vi "array -- poor man hash table -- cluster keyed .vi"(0 "key table":T2[](array[typedef]), 1 "hash key":T2, 2 "value table":T1[](array[typedef]), 3 "torque -- hash value":T1={"time (sec) array"=[], "temperature (K) array"=[], "SRS Vx (V) array"=[], "field (T) array"=[], "filename"="name", "time OK?"=FALSE, "temperature OK?"=FALSE, "SRS OK?"=FALSE, "FIELD OK?"=FALSE}, 6 "hash action":T3) -> (14 "Key table OUT":T2[](array[typedef]), 15 "hash key OUT":T2, 16 "value table OUT":T1[](array[typedef]), 17 "torque -- hash value OUT":T1={"time (sec) array"=[], "temperature (K) array"=[], "SRS Vx (V) array"=[], "field (T) array"=[], "filename"="name", "time OK?"=FALSE, "temperature OK?"=FALSE, "SRS OK?"=FALSE, "FIELD OK?"=FALSE}, 18 "index":i32, 19 "found?":bool)   [LabVIEW 2012]
uses:
  hash action control.ctl
  torque -- hash key.ctl
  torque -- hash value.ctl
  stack action -- control.ctl
  hash status control.ctl
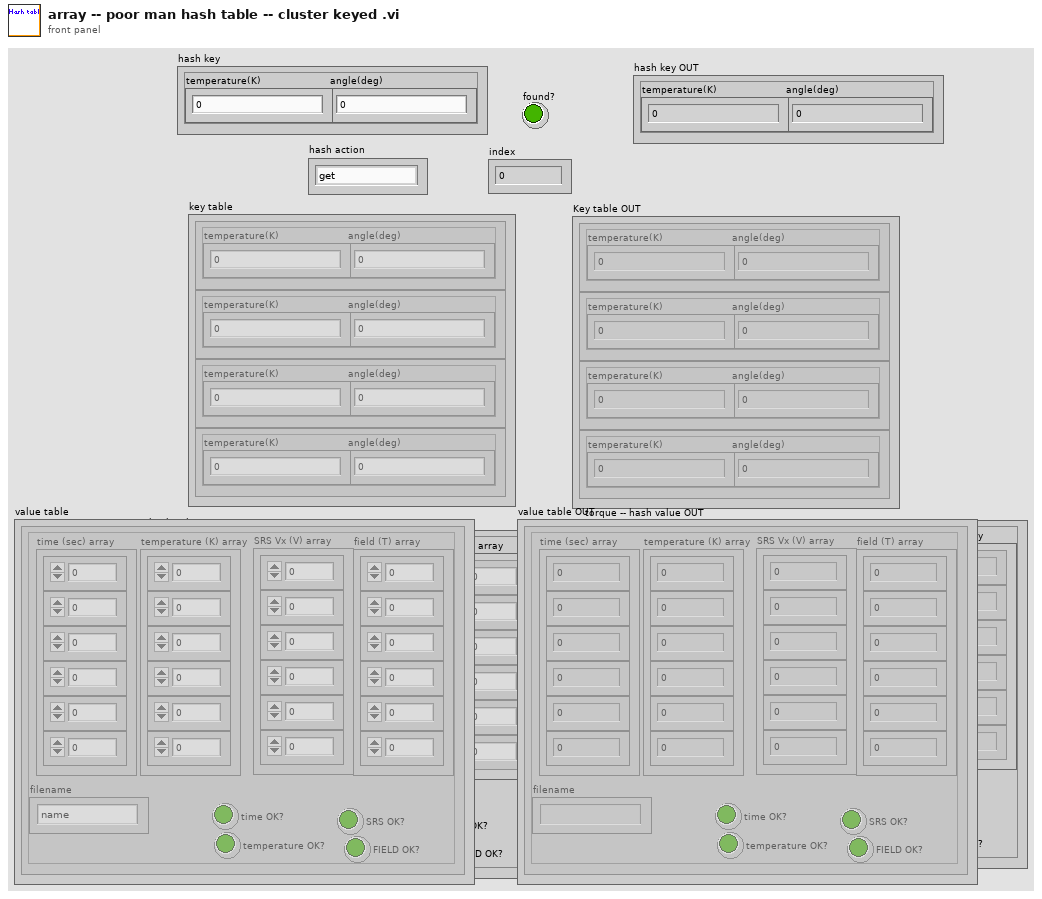
[diagram p1: front panel]
types:
  T1 = typedef "torque -- hash value.ctl" = cluster{"time (sec) array":dbl[], "temperature (K) array":dbl[], "SRS Vx (V) array":dbl[], "field (T) array":dbl[], "filename":string, "time OK?":bool, "temperature OK?":bool, "SRS OK?":bool, "FIELD OK?":bool}
  T2 = typedef "torque -- hash key.ctl" = cluster{"temperature(K)":dbl, "angle(deg)":dbl}
  T3 = typedef "hash action control.ctl" = enum16{"get", "new", "--void", "delete", "delete all", "set", "--delete if exists", "--create if not there", "list keys", "index forw", "index back", "check", "index set", "find key"}
  T4 = typedef "stack action -- control.ctl" = enum16{"push", "pop", "check", "init"}
  T5 = typedef "hash status control.ctl" = enum16{"exists", "does not exists"}
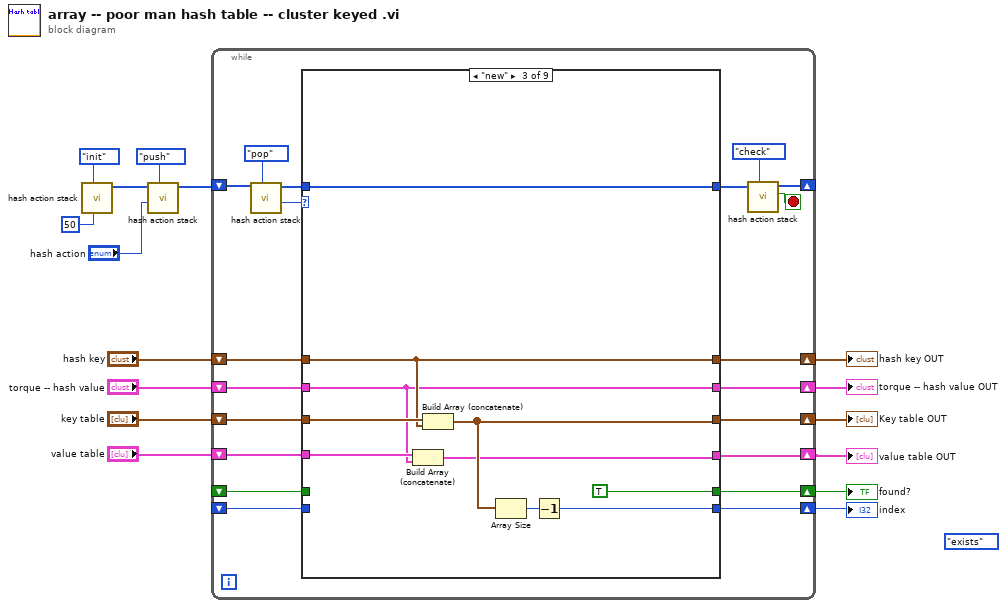
[diagram p0: block diagram]
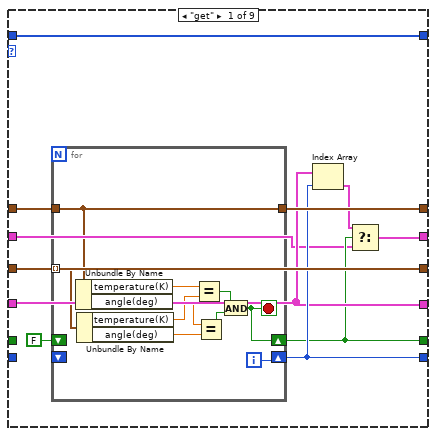
[diagram p2: hidden frame]
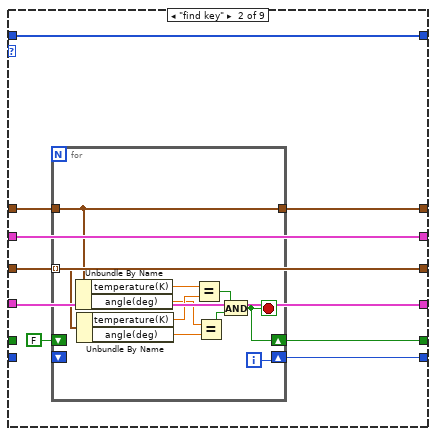
[diagram p3: hidden frame]
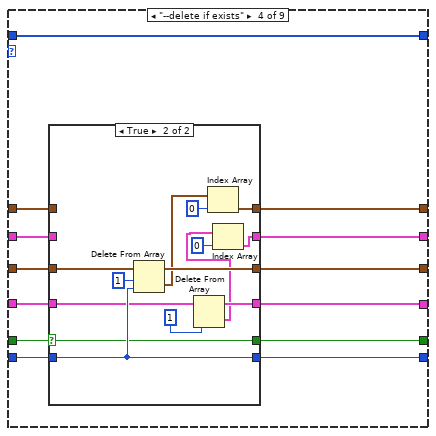
[diagram p4: hidden frame]
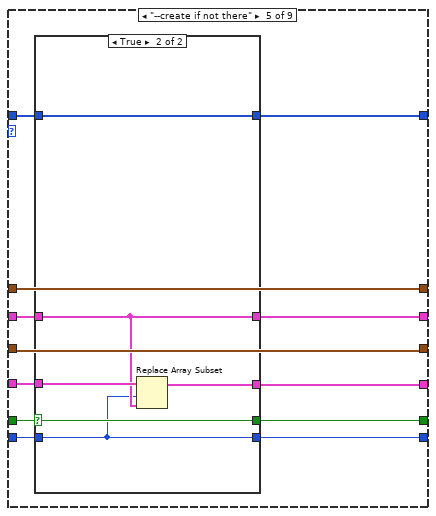
[diagram p6: hidden frame]
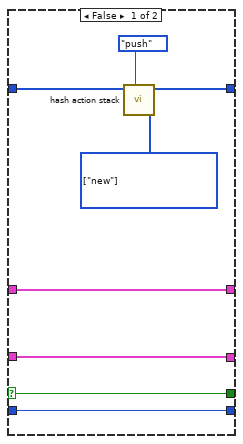
[diagram p7: hidden frame]
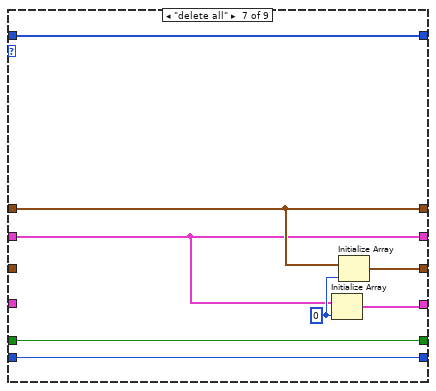
[diagram p9: hidden frame]
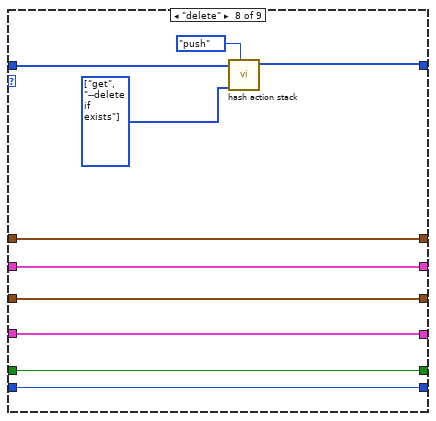
[diagram p10: hidden frame]
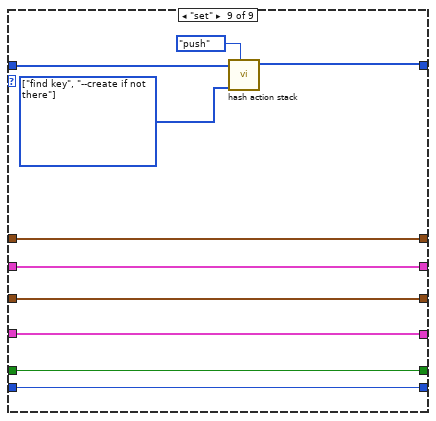
[diagram p11: hidden frame]
diagram:
  (unwired) hash_status_control."exists" ("hash status")
  n1 = call "hash action stack.vi"("init size"=50 ("dimension size"), "stack action"=stack_action_--_control."init") -> ("command stack out"=w12:T3[])  [unwired: 7 in, 2 out]
  n2 = call "hash action stack.vi"("stack action"=stack_action_--_control."push", "hash action"="hash action", "command stack"=w12) -> ("command stack out"=w14:T3[])  [unwired: 6 in, 2 out]
  n3 = while {
    shift-right: [w30] -> _
    shift-left: w14 -> [w29]
    shift-right: [w27] -> w9
    shift-left: _ -> [w21]
    shift-right: [w28] -> w10
    shift-left: _ -> [w22]
    shift-right: [w26] -> w8
    shift-left: "key table" -> [w23]
    shift-right: [w25] -> w7
    shift-left: "hash key" -> [w24]
    shift-right: [w20] -> w4
    shift-left: "torque -- hash value" -> [w18]
    shift-right: [w17] -> w3
    shift-left: "value table" -> [w19]
    stop <- w31 stop-if-true
    n4 = call "hash action stack.vi"("stack action"=stack_action_--_control."pop", "command stack"=w29) -> ("cursor window action out"=w32:T3, "command stack out"=w35:T3[])  [unwired: 7 in, 1 out]
    n5 = case shown="\"new\"" w32 {
      tunnel: w35 -> [w47 w66 w86 w99 w125 w152 w160 w164 w172]
      tunnel: [w47 w66 w86 w99 w124 w152 w160 w163 w171] -> w33
      tunnel: w23 -> [w43 w62 w85 w98 w126 w150 _ w169 w179]
      tunnel: w24 -> [w46 w65 w84 w91 w131 w151 w156 w170 w180]
      tunnel: [w40 w59 TRUE w93 w127 w149 w159 w168 w178] -> w28
      tunnel: [w42 w61 w81 w94 w128 w148 w158 w167 w177] -> w27
      tunnel: [w43 w62 w83 w97 w126 w150 w155 w169 w179] -> w26
      tunnel: [w44 w63 w84 w92 w131 w151 w156 w170 w180] -> w25
      tunnel: w22 -> [_ _ _ w95 w129 w149 w159 w168 w178]
      tunnel: w21 -> [_ _ _ w96 w130 w148 w158 w167 w177]
      tunnel: [w38 w58 w78 w90 w120 w147 w154 w162 w174] -> w20
      tunnel: w18 -> [w37 w58 w78 w89 w121 w147 w154 w162 w174]
      tunnel: w19 -> [w41 w60 w79 w87 w123 w146 _ w161 w173]
      tunnel: [w41 w60 w77 w88 w122 w146 w153 w161 w173] -> w17
      frame "get" {
        n6 = for {
          tunnel: w43 -> [w49] mode=indexing
          tunnel: w46 -> [w48]
          shift-right: [w51] -> w40
          shift-left: FALSE -> [_]
          shift-right: [w50] -> w42
          shift-left: _ -> [_]
          tunnel: [w48] -> w44
          i -> [w50]
          stop <- w51 stop-if-true
          n7 = Unbundle By Name(w48) -> ("temperature(K)"=w56:dbl, "angle(deg)"=w55:dbl)
          n8 = Unbundle By Name(w49) -> ("temperature(K)"=w57:dbl, "angle(deg)"=w54:dbl)
          n9 = Equal?(x=w56, y=w57) -> (x = y?=w53:bool)
          n10 = Equal?(x=w55, y=w54) -> (x = y?=w52:bool)
          n11 = And(x=w53, y=w52) -> (x .and. y?=w51:bool)
        }
        n12 = Index Array(array=w41, index=w42) -> (element=w39:T1)
        n13 = Select(t=w39, s=w40, f=w37) -> (s? t:f=w38:T1)
      }
      frame "find key" {
        n14 = for {
          tunnel: w62 -> [w68] mode=indexing
          tunnel: w65 -> [w67]
          shift-right: [w70] -> w59
          shift-left: FALSE -> [_]
          shift-right: [w69] -> w61
          shift-left: _ -> [_]
          tunnel: [w67] -> w63
          i -> [w69]
          stop <- w70 stop-if-true
          n15 = Unbundle By Name(w67) -> ("temperature(K)"=w75:dbl, "angle(deg)"=w74:dbl)
          n16 = Unbundle By Name(w68) -> ("temperature(K)"=w76:dbl, "angle(deg)"=w73:dbl)
          n17 = Equal?(x=w75, y=w76) -> (x = y?=w72:bool)
          n18 = Equal?(x=w74, y=w73) -> (x = y?=w71:bool)
          n19 = And(x=w72, y=w71) -> (x .and. y?=w70:bool)
        }
      }
      frame "new" {
        n20 = Build Array (concatenate)(w79, w78) -> (w77:T1[])
        n21 = Build Array (concatenate)(w85, w84) -> (w83:T2[])
        n22 = Array Size(array=w83) -> (size(s)=w82:i32)
        n23 = Decrement(x=w82) -> (x-1=w81:i32)
      }
      frame "--delete if exists" {
        n24 = case shown="True" w95 {
          selector: w95 -> [w104 w115]
          tunnel: w98 -> [w105 w119]
          tunnel: [w105 w118] -> w97
          tunnel: w96 -> [w103 w116]
          tunnel: [w103 w116] -> w94
          tunnel: [w104 w115] -> w93
          tunnel: [w102 w112] -> w92
          tunnel: w91 -> [w102 _]
          tunnel: [w101 w107] -> w90
          tunnel: w89 -> [w101 _]
          tunnel: [w100 w110] -> w88
          tunnel: w87 -> [w100 w109]
          frame False {
          }
          frame True {
            n25 = Delete From Array(array=w119, length=1, index=w116) -> (deleted portion=w114:T2[], array with subset deleted=w118:T2[])
            n26 = Delete From Array(array=w109, length=1) -> (deleted portion=w106:T1[], array with subset deleted=w110:T1[])  [unwired: 1 in]
            n27 = Index Array(array=w114, index=0) -> (element=w112:T2)
            n28 = Index Array(array=w106, index=0) -> (element=w107:T1)
          }
        }
      }
      frame "--create if not there" {
        n29 = case shown="True" w129 {
          selector: w129 -> [w138 w145]
          tunnel: w130 -> [w139 w140]
          tunnel: [w139 w140] -> w128
          tunnel: [w138 w145] -> w127
          tunnel: w125 -> [w136 w144]
          tunnel: [w135 w144] -> w124
          tunnel: w123 -> [w133 w143]
          tunnel: [w133 w142] -> w122
          tunnel: w121 -> [w134 w141]
          tunnel: [w134 w141] -> w120
          frame False {
            w132 = T3[] [enum."new"] items=["get", "new", "--void", "delete", "delete all", "set", "--delete if exists", "--create if not there", "list keys", "index forw", "index back", "check", "index set", "find key"] ("hash action list")
            n30 = call "hash action stack.vi"("stack action"=stack_action_--_control."push", "hash action list"=w132, "command stack"=w136) -> ("command stack out"=w135:T3[])  [unwired: 6 in, 2 out]
          }
          frame True {
            n31 = Replace Array Subset(array=w143, new element=w141, index=w140) -> (w142:T1[])
          }
        }
      }
      frame "--void", Default {
      }
      frame "delete all" {
        w157 = 0 ("dimension size")
        n32 = Initialize Array(w154, w157) -> (w153:T1[])
        n33 = Initialize Array(w156, w157) -> (w155:T2[])
      }
      frame "delete" {
        w165 = T3[] [enum."get", enum."--delete if exists"] items=["get", "new", "--void", "delete", "delete all", "set", "--delete if exists", "--create if not there", "list keys", "index forw", "index back", "check", "index set", "find key"] ("hash action list")
        n34 = call "hash action stack.vi"("stack action"=stack_action_--_control."push", "hash action list"=w165, "command stack"=w164) -> ("command stack out"=w163:T3[])  [unwired: 6 in, 2 out]
      }
      frame "set" {
        w175 = T3[] [enum."find key", enum."--create if not there"] items=["get", "new", "--void", "delete", "delete all", "set", "--delete if exists", "--create if not there", "list keys", "index forw", "index back", "check", "index set", "find key"] ("hash action list")
        n35 = call "hash action stack.vi"("stack action"=stack_action_--_control."push", "hash action list"=w175, "command stack"=w172) -> ("command stack out"=w171:T3[])  [unwired: 6 in, 2 out]
      }
    }
    n36 = call "hash action stack.vi"("stack action"=stack_action_--_control."check", "command stack"=w33) -> ("stack is empty ?"=w31:bool, "command stack out"=w30:T3[])  [unwired: 7 in, 1 out]
  }
  "found?" <- w10
  "index" <- w9
  "Key table OUT" <- w8
  "hash key OUT" <- w7
  "torque -- hash value OUT" <- w4
  "value table OUT" <- w3
